vi "Init.vi"(9 "Project:Active Project":refnum<vi>, 10 "NI.LV.Dialog Instance":refnum<vi>) -> (0 "error out":errorcluster, 3 "Script out":refnum<class "_Rename.lvclass">)   [LabVIEW 2020, in "_Rename.lvlib" / "_Rename.lvclass"]
uses:
  _Rename.lvclass
  _Rename.lvclass/_Rename.ctl
  <vilib>/Utility/EditLVProj/Edit LVProj.lvlib
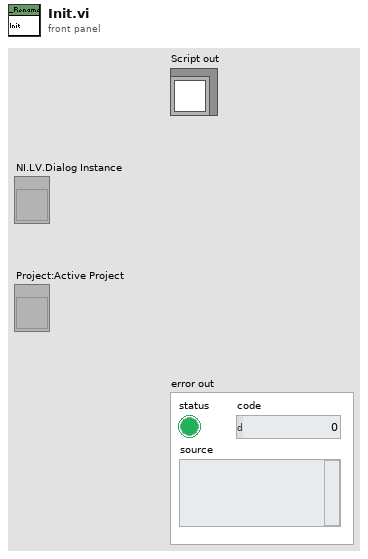
[diagram p1: front panel]
types:
  T1 = typedef "Edit LVProj.lvlib/Library And VI References.ctl" = cluster{"Target Reference":refnum<vi>, "VI References":refnum<vi>[], "Library References":refnum<vi>[]}
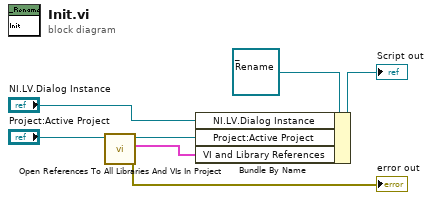
[diagram p0: block diagram]
diagram:
  n1 = call <vilib>:"Open References To All Libraries And VIs In Project.vi"("Project in"="Project:Active Project") -> ("error out"=→"error out":errorcluster, "VI and Library References"=w2:T1[], "Project out"=w3:refnum<vi>)  [unwired: 8 in]
  n2 = Bundle By Name(cluster=refnum<class "_Rename.lvclass"> refnum ("Script out"), "NI.LV.Dialog Instance"="NI.LV.Dialog Instance", "Project:Active Project"=w3, "VI and Library References"=w2) -> (→"Script out":refnum<class "_Rename.lvclass">)
